vi "x-axis.vi"(8 "error in (no error)":errorcluster, 11 "Dummy Scan in":refnum<class "Dummy Scan.lvclass">) -> (0 "error out":errorcluster, 1 "Label":string, 2 "Unit":string, 3 "Dummy Scan out":refnum<class "Dummy Scan.lvclass">)   [LabVIEW 2009, in "Dummy Scan.lvclass"]
uses:
  Dummy Scan.lvclass
  Scanner/Scanner.lvclass
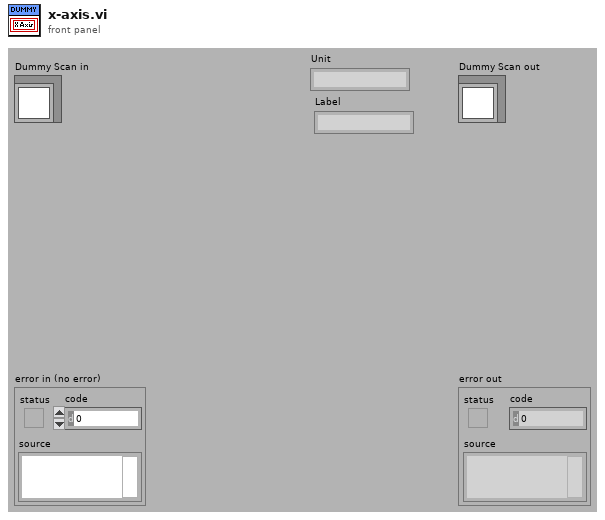
[diagram p1: front panel]
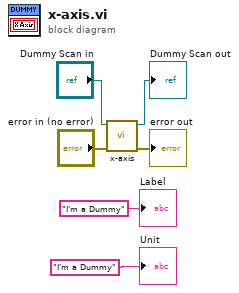
[diagram p0: block diagram]
diagram:
  n1 = call-parent "x-axis.vi"("error in (no error)"="error in (no error)", "Scanner in"="Dummy Scan in") -> ("error out"=→"error out":errorcluster, "Scanner out"=→"Dummy Scan out":refnum<class "Dummy Scan.lvclass">)  [unwired: 6 in, 2 out]
  "Label" <- "I'm a Dummy"
  "Unit" <- "I'm a Dummy"
